vi "Create New Node.vi"() -> (0 "Tree Node":refnum<data-value>)   [LabVIEW 2019]
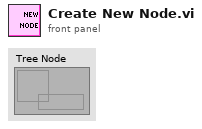
[diagram p1: front panel]
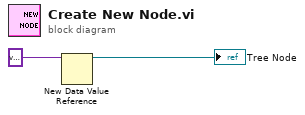
[diagram p0: block diagram]
diagram:
  n1 = New Data Value Reference(data value=variant) -> (data value reference=→"Tree Node":refnum<data-value>)  [unwired: 1 in, 1 out]
